vi "about.vi"(8 "服务器信息":T1={"host"="27.154.58.30", "port"=8020, "user"="std", "password"="std23506", "远端地址"="/微站/四代/一体化微型水质监测站.exe"}, 9 "SN输入":string="SN", 10 "站点名称输入":string="站点名称", 11 "应用程序名称输入":string="地表水水质自动监测系统") -> ()   [LabVIEW 2016, in "update.lvlib"]
uses:
  update.lvlib
  <vilib>/Utility/miscctls.llb/LVPointTypeDef.ctl
panel:
  in  "检查更新":bool
  in  "更新日志":bool
  out "SN":string="SN"
  out "站点名称":string="站点名称"
  out "Version":string="Version 1.0.0"
  out "应用程序名称":string="地表水水质自动监测系统"
  # "关于"
  # "软件名称:"
  # "软件版本:"
  # "站点名称:"
  # "序列号:"
  # "Copyright (c) 2019. All rights reserved."
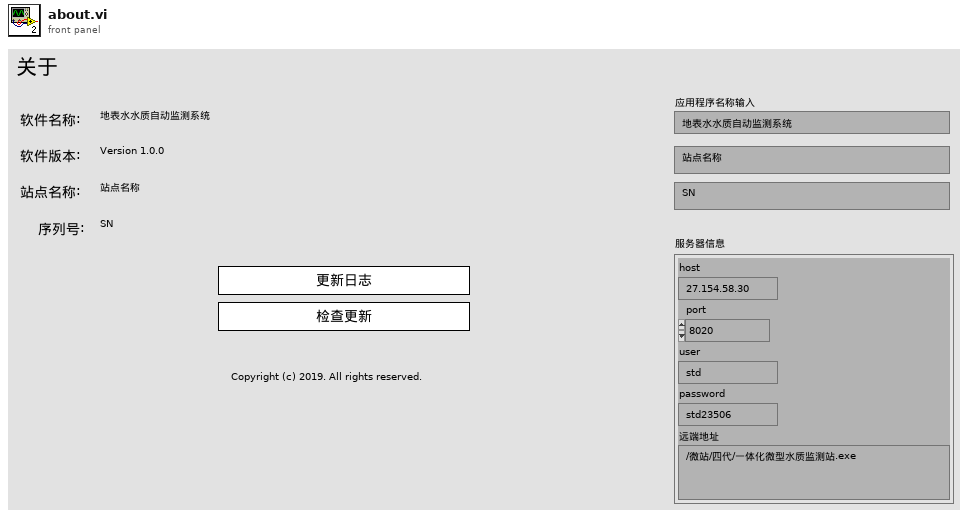
[diagram p1: front panel]
types:
  T1 = cluster{"host":string, "port":u16, "user":string, "password":string, "远端地址":string}
  T2 = typedef "LVPointTypeDef.ctl" = cluster{"Horizontal":i16, "Vertical":i16}
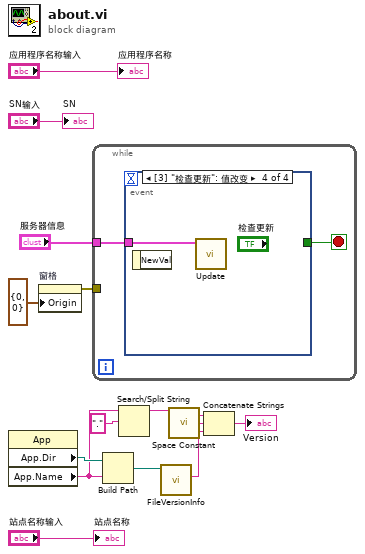
[diagram p0: block diagram]
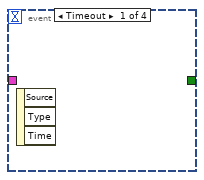
[diagram p2: hidden frame]
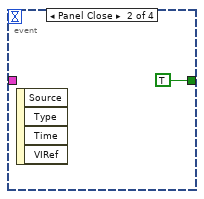
[diagram p3: hidden frame]
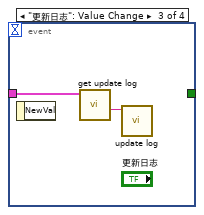
[diagram p4: hidden frame]
diagram:
  n1 = property class="App"() -> ("App.Dir"=w11:path, "App.Name"=w3:string)  [unwired: 2 in, 2 out]
  n2 = property on="窗格" class="Pane"("Origin"=T2 {"Horizontal"=0, "Vertical"=0} ("原点")) -> (error out=w13:errorcluster)  [unwired: 2 in, 1 out]
  n3 = while {
    tunnel: w13 -> [_]
    tunnel: "服务器信息" -> [w15]
    stop <- w16 stop-if-true
    n4 = event shown="[3] \"检查更新\": 值改变" {
      selector: _ -> [_ _ _ _]
      dyn-events: _ -> [_ _ _ _]
      timeout: _ -> [_ _ _ _]
      tunnel: [_ TRUE _ _] -> w16
      tunnel: w15 -> [_ _ w19 w20]
      event Timeout {
        n5 = event-data() -> ()  [unwired: 1 in, 3 out]
      }
      event Panel Close {
        n6 = event-data() -> ()  [unwired: 1 in, 4 out]
      }
      event "更新日志": Value Change {
        n7 = event-data() -> ()  [unwired: 1 in, 1 out]
        n8 = call "get update log.vi"("服务器信息"=w19) -> ("部分更新日志"=w18:string)  [unwired: 6 in, 4 out]
        n9 = call "update log.vi"("更新记录"=w18) -> ()  [unwired: 10 in, 1 out]
      }
      event "检查更新": Value Change {
        n10 = event-data() -> ()  [unwired: 1 in, 1 out]
        n11 = call "Update.vi"("服务器信息"=w20) -> ()  [unwired: 11 in]
      }
    }
  }
  n12 = Build Path(base path=w11, name or relative path=w3) -> (appended path=w10:path)
  n13 = Search/Split String(string=w3, search string/char (-)="." ("搜索字符串/字符(-)")) -> (substring before match=w1:string)  [unwired: 1 in, 2 out]
  n14 = call <vilib>:"FileVersionInfo.vi"("Application Path in"=w10) -> ("File Version Info"=w9:string)  [unwired: 7 in, 3 out]
  n15 = call <vilib>:"Space Constant.vi"() -> ("String"=w6:string)
  n16 = Concatenate Strings(w1, w6, w9) -> (→"Version":string)
  "应用程序名称" <- "应用程序名称输入"
  "站点名称" <- "站点名称输入"
  "SN" <- "SN输入"
